vi "dfd_Calculate Filter Normalization.vi"(5 "structure type":T2=enum."Lattice ARMA (basic sections)", 7 "scale type":T1=enum."Time Domain 1-Norm", 9 "coefficients a/k":dbl[](array[numeric]) format="%.2f", 10 "coefficients b/v":dbl[](array[numeric]) format="%.2f", 11 "iterations":i32) -> (2 "impulse resp":dbl[](array[numeric]), 3 "norm":dbl[](array[numeric]) format="%.2f")   [LabVIEW 2017, in "NI_DigFilter_FXP.lvlib"]
uses:
  <vilib>/addons/Digital Filter Design/NI_DigFilter_FXP.lvlib
  <vilib>/addons/Digital Filter Design/_Objects.llb/DFD Filter Structure Type Selector.ctl
  <vilib>/addons/Digital Filter Design/_Objects.llb/DFD Coef Norm Type.ctl
  <vilib>/Analysis/NI_AALBase.lvlib
  <vilib>/addons/Digital Filter Design/NI_DigFilterLicensed.lvlib
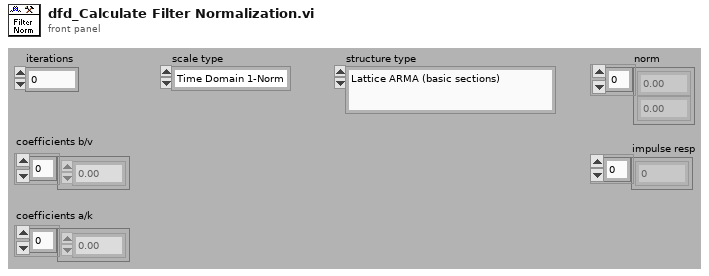
[diagram p1: front panel]
types:
  T1 = typedef "NI_DigFilterLicensed.lvlib/DFD Coef Norm Type.ctl" = enum16{"No Norm", "Time Domain 1-Norm", "Time Domain 2-Norm", "Time Domain Inf-Norm"}
  T2 = typedef "NI_DigFilterLicensed.lvlib/DFD Filter Structure Type Selector.ctl" = enum16{"Undefined", "FIR Direct Form", "FIR Direct Form Transposed", "FIR Symmetric", "FIR Antisymmetric", "IIR Direct Form I", "IIR Direct Form I Transposed", "IIR Direct Form II", "IIR Direct Form II Transposed", "IIR Cascaded Second Order Sections Form I", "IIR Cascaded Second Order Sections Form I Transposed", "IIR Cascaded Second Order Sections Form II", "IIR Cascaded Second Order Sections Form II Transposed", "Lattice Allpass (basic sections)", "Lattice Allpass (one multiplier sections)", "Lattice Allpass (normalized sections)", "Lattice AR (basic sections)", "Lattice AR (one multiplier sections)", "Lattice AR (normalized sections)", "Lattice MA (minimum phase)", "Lattice MA (maximum phase)", "Lattice ARMA (basic sections)", "Lattice ARMA (one multiplier sections)", "Lattice ARMA (normalized sections)"}
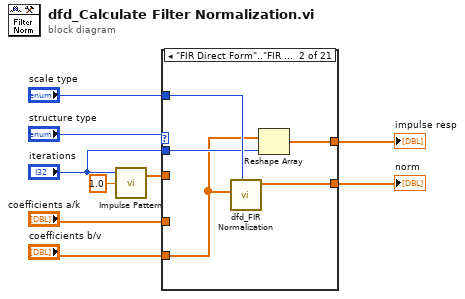
[diagram p0: block diagram]
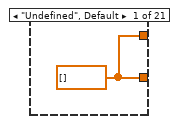
[diagram p2: hidden frame]
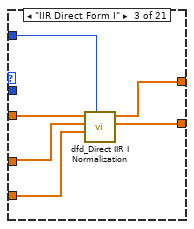
[diagram p3: hidden frame]
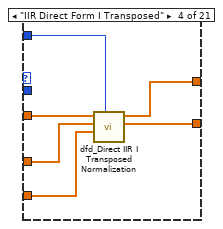
[diagram p4: hidden frame]
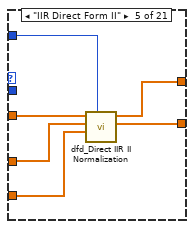
[diagram p5: hidden frame]
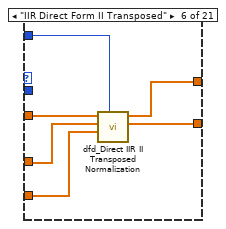
[diagram p6: hidden frame]
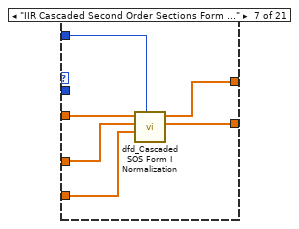
[diagram p7: hidden frame]
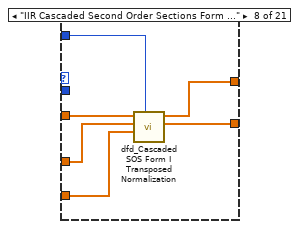
[diagram p8: hidden frame]
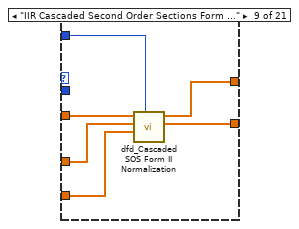
[diagram p9: hidden frame]
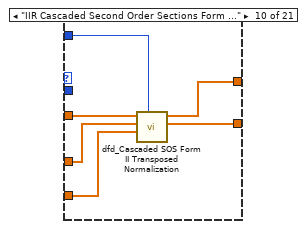
[diagram p10: hidden frame]
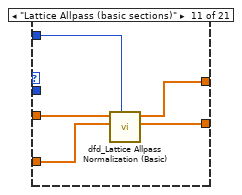
[diagram p11: hidden frame]
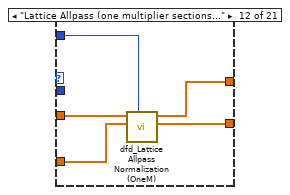
[diagram p12: hidden frame]
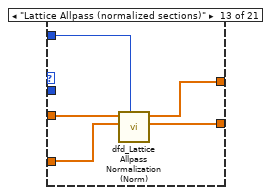
[diagram p13: hidden frame]
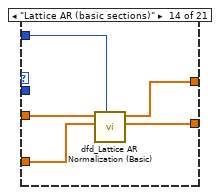
[diagram p14: hidden frame]
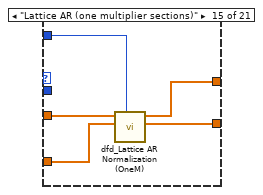
[diagram p15: hidden frame]
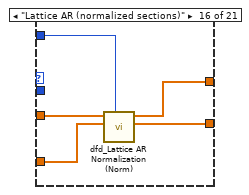
[diagram p16: hidden frame]
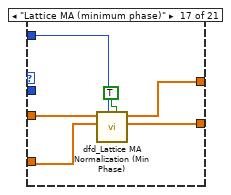
[diagram p17: hidden frame]
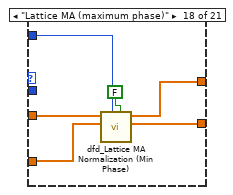
[diagram p18: hidden frame]
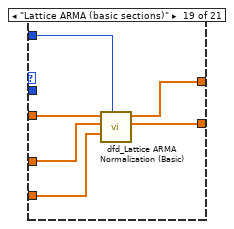
[diagram p19: hidden frame]
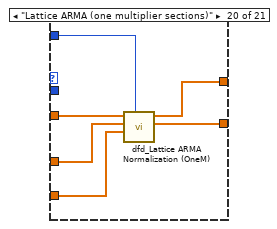
[diagram p20: hidden frame]
diagram:
  n1 = call <vilib>:"Impulse Pattern.vi"("amplitude"=1.0, "samples"="iterations") -> ("Impulse Pattern"=w4:dbl[])  [unwired: 1 in, 1 out]
  n2 = case shown="\"FIR Direct Form\"..\"FIR Antisymmetric\"" "structure type" {
    tunnel: "coefficients b/v" -> [_ w12 w19 w24 w30 w36 w43 w49 w54 w60 _ _ _ _ _ _ _ _ w108 w114 w121]
    tunnel: [w10 w14 w17 w23 w29 w35 w41 w47 w53 w59 w65 w70 w75 w80 w85 w90 w95 w101 w107 w113 w119] -> w7
    tunnel: "coefficients a/k" -> [_ _ w20 w25 w31 w37 w44 w50 w55 w61 w68 w72 w77 w82 w87 w91 w97 w105 w109 w115 w122]
    tunnel: w4 -> [_ _ w21 w27 w33 w39 w45 w51 w57 w63 w67 w73 w78 w83 w88 w93 w99 w102 w111 w117 w123]
    tunnel: "scale type" -> [_ w15 w18 w26 w32 w38 w42 w48 w56 w62 w66 w71 w76 w81 w86 w92 w98 w104 w110 w116 w120]
    tunnel: "iterations" -> [_ w13 _ _ _ _ _ _ _ _ _ _ _ _ _ _ _ _ _ _ _]
    tunnel: [w10 w11 w16 w22 w28 w34 w40 w46 w52 w58 w64 w69 w74 w79 w84 w89 w94 w100 w106 w112 w118] -> w1
    frame "Undefined", Default {
      w10 = dbl[] [] ("norm")
    }
    frame "FIR Direct Form".."FIR Antisymmetric" {
      n3 = call <vilib>:"dfd_FIR Normalization.vi"("scale type"=w15, "coeffcients b"=w12) -> ("norm"=w14:dbl[])  [unwired: 9 out]
      n4 = Reshape Array(w12, w13) -> (w11:dbl[])
    }
    frame "IIR Direct Form I" {
      n5 = call <vilib>:"dfd_Direct IIR I Normalization.vi"("scale type"=w18, "coefficients b"=w19, "coefficients a"=w20, "x"=w21) -> ("norm"=w17:dbl[], "y"=w16:dbl[])  [unwired: 6 out]
    }
    frame "IIR Direct Form I Transposed" {
      n6 = call <vilib>:"dfd_Direct IIR I Transposed Normalization.vi"("scale type"=w26, "coefficients b"=w24, "coefficients a"=w25, "x"=w27) -> ("norm"=w23:dbl[], "y"=w22:dbl[])  [unwired: 6 out]
    }
    frame "IIR Direct Form II" {
      n7 = call <vilib>:"dfd_Direct IIR II Normalization.vi"("scale type"=w32, "coefficients b"=w30, "coefficients a"=w31, "x"=w33) -> ("norm"=w29:dbl[], "y"=w28:dbl[])  [unwired: 6 out]
    }
    frame "IIR Direct Form II Transposed" {
      n8 = call <vilib>:"dfd_Direct IIR II Transposed Normalization.vi"("scale type"=w38, "coefficients b"=w36, "coefficients a"=w37, "x"=w39) -> ("norm"=w35:dbl[], "y"=w34:dbl[])  [unwired: 6 out]
    }
    frame "IIR Cascaded Second Order Sections Form I" {
      n9 = call <vilib>:"dfd_Cascaded SOS Form I Normalization.vi"("scale type"=w42, "coefficients b"=w43, "coefficients a"=w44, "x"=w45) -> ("norm"=w41:dbl[], "y"=w40:dbl[])  [unwired: 6 out]
    }
    frame "IIR Cascaded Second Order Sections Form I Transposed" {
      n10 = call <vilib>:"dfd_Cascaded SOS Form I Transposed Normalization.vi"("scale type"=w48, "coefficients b"=w49, "coefficients a"=w50, "x"=w51) -> ("norm"=w47:dbl[], "y"=w46:dbl[])  [unwired: 6 out]
    }
    frame "IIR Cascaded Second Order Sections Form II" {
      n11 = call <vilib>:"dfd_Cascaded SOS Form II Normalization.vi"("scale type"=w56, "coefficients b"=w54, "coefficients a"=w55, "x"=w57) -> ("norm"=w53:dbl[], "y"=w52:dbl[])  [unwired: 6 out]
    }
    frame "IIR Cascaded Second Order Sections Form II Transposed" {
      n12 = call <vilib>:"dfd_Cascaded SOS Form II Transposed Normalization.vi"("scale type"=w62, "coefficients b"=w60, "coefficients a"=w61, "x"=w63) -> ("norm"=w59:dbl[], "y"=w58:dbl[])  [unwired: 6 out]
    }
    frame "Lattice Allpass (basic sections)" {
      n13 = call <vilib>:"dfd_Lattice Allpass Normalization (Basic).vi"("scale type"=w66, "coefficients k"=w68, "x"=w67) -> ("norm"=w65:dbl[], "y"=w64:dbl[])  [unwired: 7 out]
    }
    frame "Lattice Allpass (one multiplier sections)" {
      n14 = call <vilib>:"dfd_Lattice Allpass Normalization (OneM).vi"("scale type"=w71, "coefficients k"=w72, "x"=w73) -> ("norm"=w70:dbl[], "y"=w69:dbl[])  [unwired: 7 out]
    }
    frame "Lattice Allpass (normalized sections)" {
      n15 = call <vilib>:"dfd_Lattice Allpass Normalization (Norm).vi"("scale type"=w76, "coefficients k"=w77, "x"=w78) -> ("norm"=w75:dbl[], "y"=w74:dbl[])  [unwired: 7 out]
    }
    frame "Lattice AR (basic sections)" {
      n16 = call <vilib>:"dfd_Lattice AR Normalization (Basic).vi"("scale type"=w81, "coefficients k"=w82, "x"=w83) -> ("norm"=w80:dbl[], "y"=w79:dbl[])  [unwired: 7 out]
    }
    frame "Lattice AR (one multiplier sections)" {
      n17 = call <vilib>:"dfd_Lattice AR Normalization (OneM).vi"("scale type"=w86, "coefficients k"=w87, "x"=w88) -> ("norm"=w85:dbl[], "y"=w84:dbl[])  [unwired: 7 out]
    }
    frame "Lattice AR (normalized sections)" {
      n18 = call <vilib>:"dfd_Lattice AR Normalization (Norm).vi"("scale type"=w92, "coefficients k"=w91, "x"=w93) -> ("norm"=w90:dbl[], "y"=w89:dbl[])  [unwired: 7 out]
    }
    frame "Lattice MA (minimum phase)" {
      n19 = call <vilib>:"dfd_Lattice MA Normalization (Min Phase).vi"("min?"=TRUE, "scale type"=w98, "coefficients k"=w97, "x"=w99) -> ("norm"=w95:dbl[], "y"=w94:dbl[])  [unwired: 6 out]
    }
    frame "Lattice MA (maximum phase)" {
      n20 = call <vilib>:"dfd_Lattice MA Normalization (Min Phase).vi"("min?"=FALSE, "scale type"=w104, "coefficients k"=w105, "x"=w102) -> ("norm"=w101:dbl[], "y"=w100:dbl[])  [unwired: 6 out]
    }
    frame "Lattice ARMA (basic sections)" {
      n21 = call <vilib>:"dfd_Lattice ARMA Normalization (Basic).vi"("scale type"=w110, "coefficients v"=w108, "coefficients k"=w109, "x"=w111) -> ("norm"=w107:dbl[], "y"=w106:dbl[])  [unwired: 6 out]
    }
    frame "Lattice ARMA (one multiplier sections)" {
      n22 = call <vilib>:"dfd_Lattice ARMA Normalization (OneM).vi"("scale type"=w116, "coefficients v"=w114, "coefficients k"=w115, "x"=w117) -> ("norm"=w113:dbl[], "y"=w112:dbl[])  [unwired: 6 out]
    }
    frame "Lattice ARMA (normalized sections)" {
      n23 = call <vilib>:"dfd_Lattice ARMA Normalization (Norm).vi"("scale type"=w120, "coefficients v"=w121, "coefficients k"=w122, "x"=w123) -> ("norm"=w119:dbl[], "y"=w118:dbl[])  [unwired: 6 out]
    }
  }
  "norm" <- w7
  "impulse resp" <- w1
